vi "Balanced_Accuracy_Score.vi"(8 "error in (no error)":errorcluster caption="entrée d'erreur (pas d'erreur)", 9 "y_pred":string[][](array[string]), 10 "y_true":string[][](array[string]), 11 "balanced_accuracy_score":cluster{"sample_weight":dbl[], "adjusted":bool}) -> (0 "error out":errorcluster caption="sortie d'erreur", 3 "Score":string)   [LabVIEW 2020]
doc: "Compute the balanced accuracy\n\nThe balanced accuracy in binary and multiclass classification problems to deal with imbalanced datasets. It is defined as the average of recall obtained on each class.\n\nThe best value is 1 and the worst value is 0 when adjusted=False.\n\n\nParameters : \n\n- y_true : 1d array-like\nGround truth (correct) target values.\n\n- y_pred : 1d array-like\nEstimated targets as returned by a classifier.\n\n- sample_weight : array-like of shape (n_samples,), default=None\nSample weights.\n\n- adjusted : bool, default=False\nWhen true, the result is adjusted for chance, so that random performance would score 0, and perfect performance scores 1.\n\nReturns : \n\n- balanced_accuracy : float"
uses:
  Balanced_Accuracy_Score.lvclass
panel:
  out "Balanced_Accuracy_Score.lvclass":refnum<class "Balanced_Accuracy_Score.lvclass">
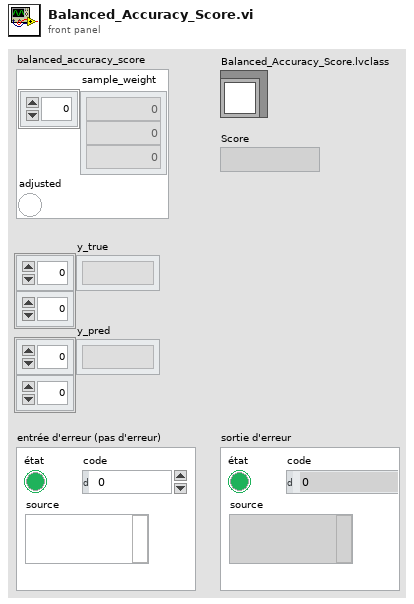
[diagram p1: front panel]
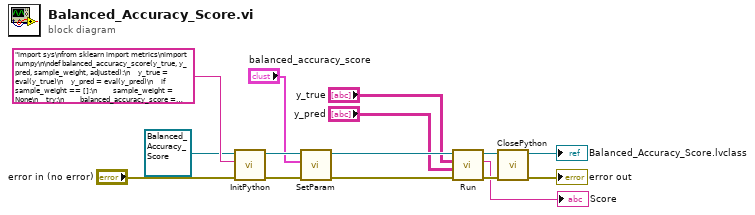
[diagram p0: block diagram]
diagram:
  n1 = call-dynamic "InitPython.vi"("error in (no error)"="error in (no error)", "Python Instruction"="import sys\nfrom sklearn import metrics\nimport numpy\n\ndef balanced_accuracy_score(y_true, y_pred, sample_weight, adjusted):\n    y_true = eval(y_true)\n    y_pred = eval(y_pred)\n    if sample_weight == []:\n        sample_weight = None\n    try:\n        balanced_accuracy_score = metrics.balanced_accuracy_score(y_true, y_pred, sample_weight, adjusted)\n        balanced_accuracy_score = balanced_accuracy_score.tolist()\n        return str(balanced_accuracy_score)\n    except:\n        erreur = sys.exc_info()\n        typerr = u\"%s\" % (erreur[0])\n        typerr = typerr[typerr.find(\"'\")+1:typerr.rfind(\"'\")]\n        msgerr = u\"%s\" % (erreur[1])\n        message = str('/!\\\\ {0} : {1}'. format(typerr,msgerr))\n        return message", "Scikit-learn en entrée"=refnum<class "Balanced_Accuracy_Score.lvclass"> refnum ("Balanced_Accuracy_Score.lvclass")) -> ("error out"=w12:errorcluster, "Scikit-learn en sortie"=w10:refnum<class "Balanced_Accuracy_Score.lvclass">)  [unwired: 7 in]
  n2 = call-dynamic "SetParam.vi"("error in (no error)"=w12, "balanced_accuracy_score"="balanced_accuracy_score", "Balanced_Accuracy_Score.lvclass"=w10) -> ("error out"=w7:errorcluster, "Balanced_Accuracy_Score.lvclass"=w8:refnum<class "Balanced_Accuracy_Score.lvclass">)  [unwired: 7 in]
  n3 = call-dynamic "Run.vi"("error in (no error)"=w7, "y_pred"="y_pred", "y_true"="y_true", "Balanced_Accuracy_Score.lvclass"=w8) -> ("error out"=w5:errorcluster, "Score"=→"Score":string, "Balanced_Accuracy_Score.lvclass"=w6:refnum<class "Balanced_Accuracy_Score.lvclass">)  [unwired: 5 in]
  n4 = call-dynamic "ClosePython.vi"("error in (no error)"=w5, "Scikit-learn en entrée"=w6) -> ("error out"=→"error out":errorcluster, "Scikit-learn en sortie"=→"Balanced_Accuracy_Score.lvclass":refnum<class "Balanced_Accuracy_Score.lvclass">)  [unwired: 8 in]
